vi "Set State Controls.vi"(7 "활성화 (F)":bool, 8 "error in (no error)":errorcluster caption="에러 입력(에러 없음)", 11 "컨트롤 참조 배열 in":refnum<vi>[](array[refnum])) -> (0 "error out":errorcluster caption="에러 출력", 3 "컨트롤 참조 배열 out":refnum<vi>[](array[refnum]))   [LabVIEW 2020]
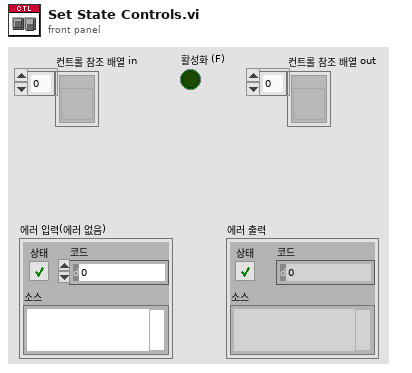
[diagram p1: front panel]
types:
  T1 = enum8{"Enabled", "Disabled", "Disabled and Grayed Out"}
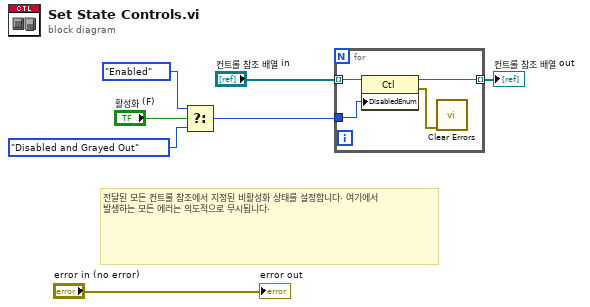
[diagram p0: block diagram]
diagram:
  # "전달된 모든 컨트롤 참조에서 지정된 비활성화 상태를 설정합니다. 여기에서 발생하는 모든 에러는 의도적으로 무시됩니다."
  n1 = Select(t=T1."Enabled" ("비활성화"), s="활성화 (F)", f=T1."Disabled and Grayed Out" ("비활성화")) -> (s? t:f=w2:T1)
  n2 = for {
    tunnel: w2 -> [w10]
    tunnel: "컨트롤 참조 배열 in" -> [w11] mode=indexing
    tunnel: [w9] -> w6 mode=indexing
    n3 = property on="프로퍼티 노드" class="Ctl"(reference=w11, "DisabledEnum"=w10) -> (reference out=w9:refnum<vi>, error out=w8:errorcluster)  [unwired: 1 in]
    n4 = call <vilib>:"Clear Errors.vi"("error in (no error)"=w8) -> ()  [unwired: 5 in, 2 out]
  }
  "컨트롤 참조 배열 out" <- w6
  "error out" <- "error in (no error)"
